vi "checkFinishPrepareKickoffEnemyPlay.vi"(8 "error in (no error)":errorcluster, 9 "last command_interpreted":T1, 10 "Game":refnum<class "Game.lvclass">, 11 "PrepareKickoffEnemyPlay in":refnum<class "PrepareKickoffEnemyPlay.lvclass">) -> (0 "error out":errorcluster, 2 "Boolean":bool, 3 "PrepareKickoffEnemyPlay out":refnum<class "PrepareKickoffEnemyPlay.lvclass">)   [LabVIEW 2023, in "PrepareKickoffEnemyPlay.lvclass"]
uses:
  PrepareKickoffEnemyPlay.lvclass
  Game_class/Game.lvclass
  Referee_class/command_interpreted.ctl
  Game_class/Game.lvclass/Game.ctl
  Referee_class/Referee.lvclass/Referee.ctl
  Events_class/Events.lvclass/Events.ctl
  Game_class/Read Referee.vi
  Game_class/Read EventsRef.vi
  Events_class/Read kick.vi
  Events_class/Read ball_out.vi
  Referee_class/Read command_interpreted.vi
  Referee_class/Referee.lvclass
  Events_class/Events.lvclass
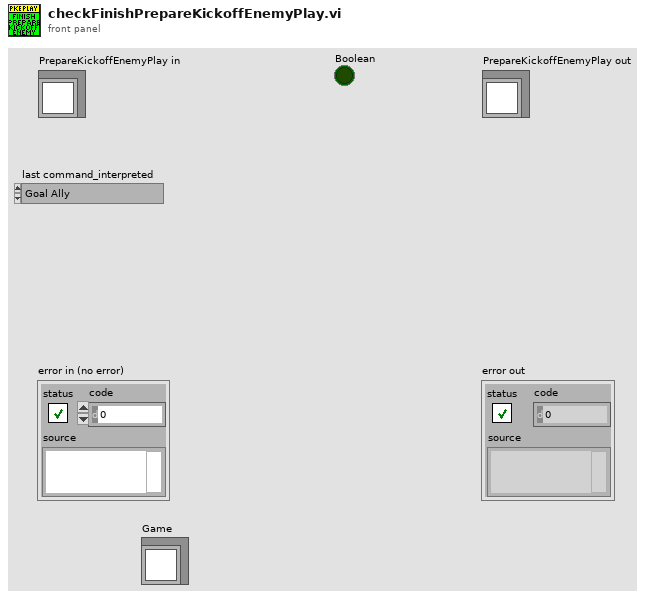
[diagram p1: front panel]
types:
  T1 = typedef "command_interpreted.ctl" = enum16{"Goal Ally", "Goal Enemy", "Ball Placement Enemy", "Ball Placement Ally", "Normal Half Time", "Extra Time  Break", "Extra Half Time", "None", "Post Game", "PKA Normal Start", "Prepare Kickoff Ally", "PKE Normal Start", "Prepare Kickoff Enemy", "Force Start", "Halt", "Timeout", "Prepare Penalty Ally", "Prepare Penalty Enemy", "PPA NormalStart", "PPE Normal Start", "Indirect Free Ally", "Direct Free Enemy", "Direct Free Ally", "Indirect Free Enemy", "Stop"}
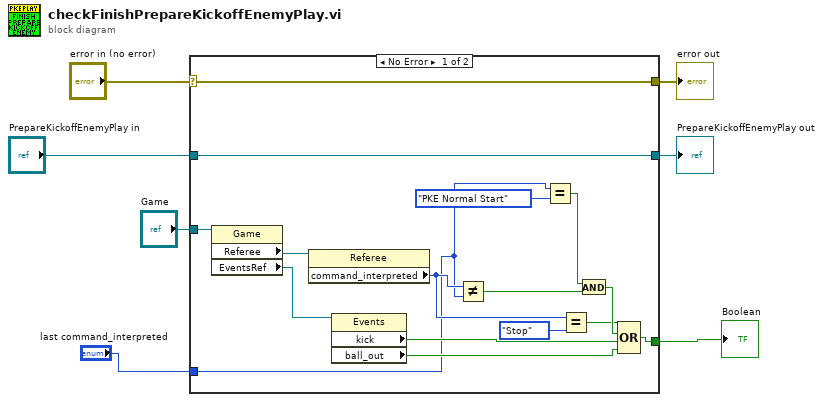
[diagram p0: block diagram]
diagram:
  n1 = case shown="No Error" "error in (no error)" {
    selector: "error in (no error)" -> [w22 w25]
    tunnel: [w22 w25] -> w6
    tunnel: [w23 w24] -> w4
    tunnel: "PrepareKickoffEnemyPlay in" -> [w23 w24]
    tunnel: "Game" -> [w17 _]
    tunnel: [w12 _] -> w2
    tunnel: "last command_interpreted" -> [w8 _]
    frame No Error {
      n2 = property class="Game"(reference=w17) -> ("Referee"=w21:refnum<class "Referee.lvclass">, "EventsRef"=w16:refnum<class "Events.lvclass">)  [unwired: 1 in, 2 out]
      n3 = property class="Referee"(reference=w21) -> ("command_interpreted"=w10:T1)  [unwired: 1 in, 2 out]
      n4 = property class="Events"(reference=w16) -> ("kick"=w14:bool, "ball_out"=w13:bool)  [unwired: 1 in, 2 out]
      n5 = Not Equal?(x=w10, y=w8) -> (x != y?=w18:bool)
      n6 = Equal?(x=w8, y=command_interpreted."PKE Normal Start" ("command_interpreted")) -> (x = y?=w19:bool)
      n7 = Equal?(x=w10, y=command_interpreted."Stop" ("command_interpreted")) -> (x = y?=w11:bool)
      n8 = And(x=w19, y=w18) -> (x .and. y?=w15:bool)
      n9 = Compound Arithmetic op=OR(w11, w15, w14, w13) -> (w12:bool)
    }
    frame Error {
    }
  }
  "error out" <- w6
  "PrepareKickoffEnemyPlay out" <- w4
  "Boolean" <- w2
